vi "GV_Zoom_StackSize.vi"(5 "Boolean-id":bool[](array[boolean]), 7 "AutoScale":T1, 9 "Graph-ref":refnum<vi>, 11 "BooleanPixels":u16) -> (1 "Bottoms":dbl[](array[numeric]), 3 "Tops":dbl[](array[numeric]))   [LabVIEW 2020, in "Sgraph_lib_V1.lvlib" / "Gviewer.lvclass"]
doc: "Determine the stack sizes for a combination of numerical and boolean tags,\nwhen some kind of stacked autoscale is used."
uses:
  Gviewer.lvclass
  controls/AutoScale.ctl
  <vilib>/Utility/miscctls.llb/LVPoint32TypeDef.ctl
panel:
  out "Error OUT":errorcluster
  in  "error in (no error)":errorcluster
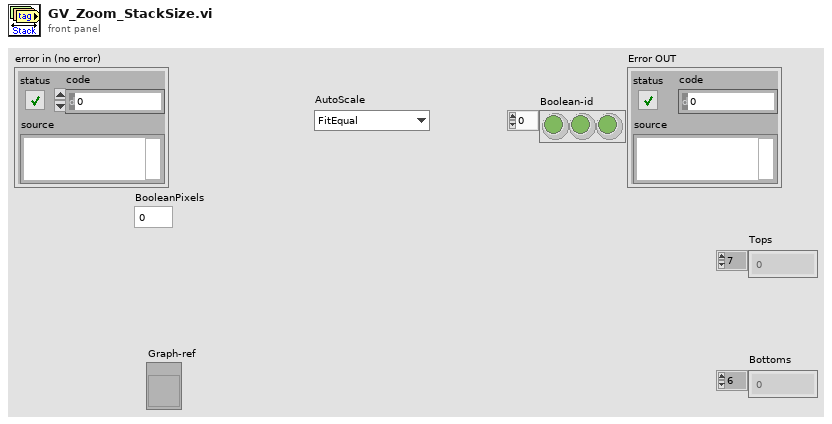
[diagram p1: front panel]
types:
  T1 = typedef "Sgraph_lib_V1.lvlib/Gviewer.lvclass/AutoScale.ctl" = enum16{"FitEqual", "FitMax", "StackEqual", "StackMax", "StackPerType"}
  T2 = typedef "LVPoint32TypeDef.ctl" = cluster{"Horizontal":i32, "Vertical":i32}
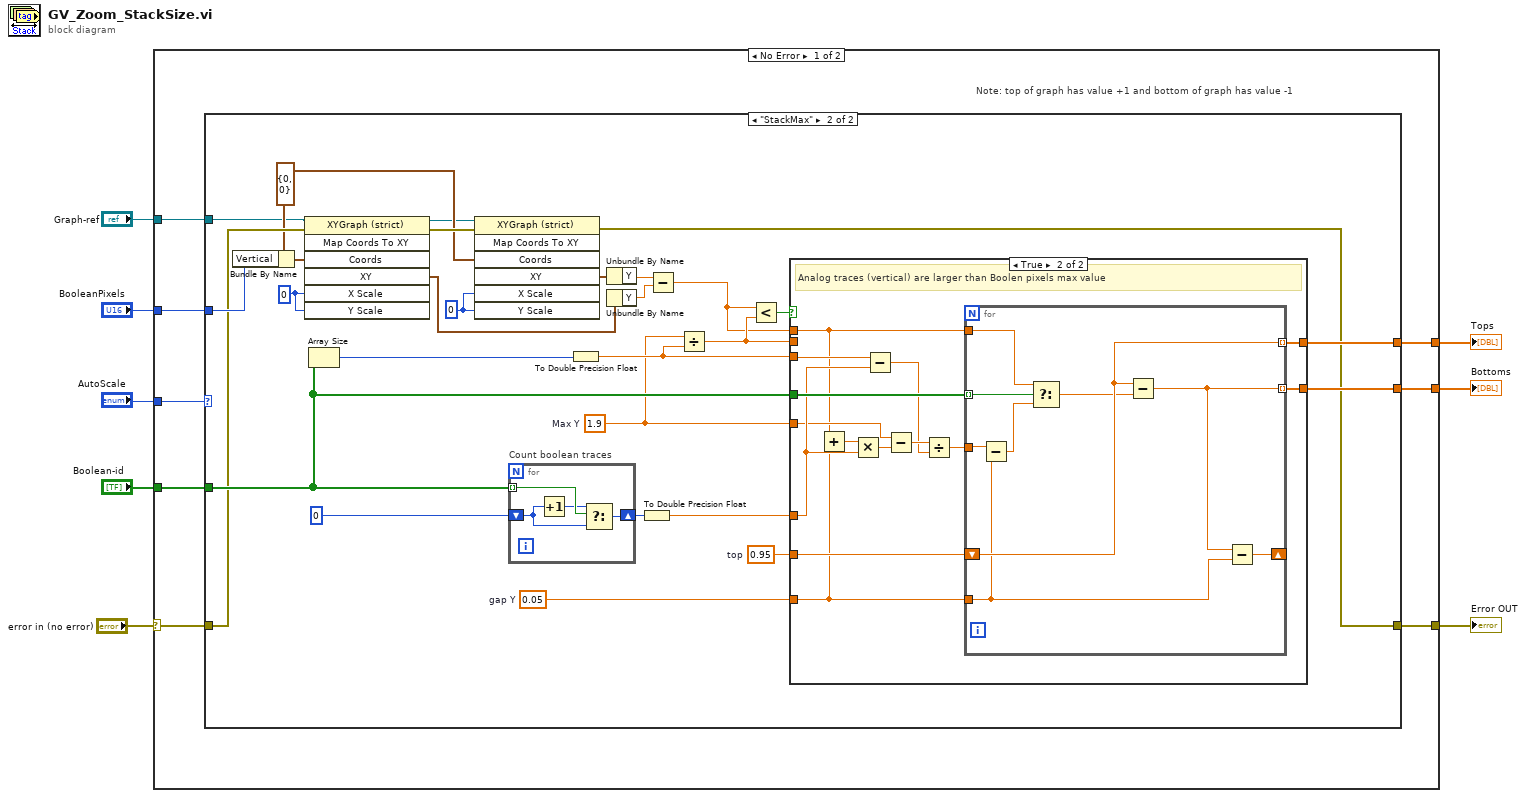
[diagram p0: block diagram]
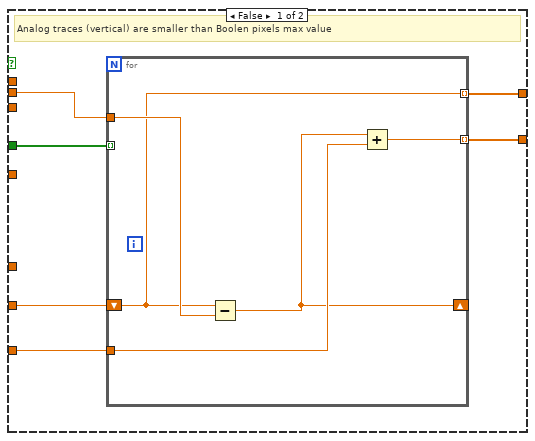
[diagram p3: hidden frame]
diagram:
  n1 = case shown="No Error" "error in (no error)" {
    selector: "error in (no error)" -> [w12 w84]
    tunnel: "Boolean-id" -> [w16 _]
    tunnel: "AutoScale" -> [w15 _]
    tunnel: "BooleanPixels" -> [w14 _]
    tunnel: "Graph-ref" -> [w13 _]
    tunnel: [w11 w84] -> w3
    tunnel: [w10 _] -> w2
    tunnel: [w9 _] -> w1
    frame No Error {
      # "Note: top of graph has value +1 and bottom of graph has value -1"
      n2 = case shown="\"StackMax\"" w15 {
        tunnel: w16 -> [_ w35]
        tunnel: w14 -> [_ w33]
        tunnel: w13 -> [_ w19]
        tunnel: w12 -> [w17 w29]
        tunnel: [w17 w30] -> w11
        tunnel: [_ w41] -> w10
        tunnel: [_ w40] -> w9
        frame Default {
        }
        frame "StackMax" {
          w20 = 0 ("X Scale")
          w32 = 0.95  # top
          w27 = T2 {"Horizontal"=0, "Vertical"=0} ("Coords")
          w42 = 0.05  # gap Y
          w31 = 1.9  # Max Y
          w21 = 0 ("X Scale")
          n3 = Bundle By Name(cluster=w27, "Vertical"=w33) -> (w26:T2)
          n4 = invoke class="XYGraph (strict)" method="Map Coords To XY"(reference=w19, error in=w29, "Coords"=w26, "X Scale"=w21, "Y Scale"=w21) -> (reference out=w18:refnum<vi>, error out=w28:errorcluster, "XY"=w25:cluster{"X":dbl, "Y":dbl})  [unwired: 2 in, 4 out]
          n5 = Array Size(array=w35) -> (size(s)=w38:i32)
          n6 = invoke class="XYGraph (strict)" method="Map Coords To XY"(reference=w18, error in=w28, "Coords"=w27, "X Scale"=w20, "Y Scale"=w20) -> (error out=w30:errorcluster, "XY"=w44:cluster{"X":dbl, "Y":dbl})  [unwired: 2 in, 5 out]
          n7 = for "Count boolean traces" {
            tunnel: w35 -> [w83] mode=indexing
            shift-right: [w80] -> w39
            shift-left: 0 ("y") -> [w82]
            n8 = Increment(x=w82) -> (x+1=w81:i32)
            n9 = Select(t=w81, s=w83, f=w82) -> (s? t:f=w80:i32)
          }
          n10 = To Double Precision Float(number=w38) -> (double precision float=w37:dbl)
          n11 = Unbundle By Name(w44) -> ("Y"=w24:dbl)
          n12 = Unbundle By Name(w25) -> ("Y"=w23:dbl)
          n13 = To Double Precision Float(number=w39) -> (double precision float=w34:dbl)
          n14 = Subtract(x=w24, y=w23) -> (x-y=w22:dbl)
          n15 = Divide(x=w31, y=w37) -> (x/y=w36:dbl)
          n16 = Less?(x=w22, y=w36) -> (x < y?=w43:bool)
          n17 = case shown="True" w43 {
            tunnel: w42 -> [w51 w58]
            tunnel: [w50 w70] -> w41
            tunnel: [w49 w69] -> w40
            tunnel: w32 -> [w48 w67]
            tunnel: w37 -> [_ w64]
            tunnel: w22 -> [_ w59]
            tunnel: w36 -> [w47 _]
            tunnel: w35 -> [w46 w68]
            tunnel: w34 -> [_ w61]
            tunnel: w31 -> [_ w60]
            frame False {
              # "Analog traces (vertical) are smaller than Boolen pixels max value"
              n18 = for {
                tunnel: w51 -> [w54]
                tunnel: [w55] -> w50 mode=indexing
                tunnel: [w52] -> w49 mode=indexing
                shift-right: [w53] -> _
                shift-left: w48 -> [w55]
                tunnel: w47 -> [w56]
                tunnel: w46 -> [_] mode=indexing
                n19 = Subtract(x=w55, y=w56) -> (x-y=w53:dbl)
                n20 = Add(x=w53, y=w54) -> (x+y=w52:dbl)
              }
            }
            frame True {
              # "Analog traces (vertical) are larger than Boolen pixels max value"
              n21 = Add(x=w59, y=w58) -> (x+y=w57:dbl)
              n22 = Multiply(x=w57, y=w61) -> (x*y=w66:dbl)
              n23 = Subtract(x=w64, y=w61) -> (x-y=w63:dbl)
              n24 = Subtract(x=w60, y=w66) -> (x-y=w65:dbl)
              n25 = Divide(x=w65, y=w63) -> (x/y=w62:dbl)
              n26 = for {
                tunnel: w58 -> [w72]
                tunnel: [w78] -> w70 mode=indexing
                tunnel: [w75] -> w69 mode=indexing
                shift-right: [w74] -> _
                shift-left: w67 -> [w78]
                tunnel: w68 -> [w79] mode=indexing
                tunnel: w62 -> [w73]
                tunnel: w59 -> [w76]
                n27 = Subtract(x=w73, y=w72) -> (x-y=w71:dbl)
                n28 = Select(t=w76, s=w79, f=w71) -> (s? t:f=w77:dbl)
                n29 = Subtract(x=w78, y=w77) -> (x-y=w75:dbl)
                n30 = Subtract(x=w75, y=w72) -> (x-y=w74:dbl)
              }
            }
          }
        }
      }
    }
    frame Error {
    }
  }
  "Tops" <- w2
  "Bottoms" <- w1
  "Error OUT" <- w3
